vi "expt_controller.vi"() -> ()   [LabVIEW 2019]
uses:
  Quantum Composers 9000 Series/Public/Configure/Configure Chan Mode (Normal).vi
  Quantum Composers 9000 Series/Quantum Composers 9000 Series.lvlib
panel:
  in  "Save condtions":bool=TRUE
  in  "Tab Control":T1(tab)
  in  "Target translation / V":dbl
  in  "Target rotation / V":dbl
  in  "Float / V":dbl
  in  "Q-switch delay / us":dbl
  in  "Delay (rel to gas pulse) / us":dbl
  in  "Gas pulse enable":bool
  in  "Ablation Laser Enable":bool
  in  "stop":bool
  in  "stop 2":bool
  in  "Tab Control 2":enum32{"Ion Optics", "Gas Controls"}(tab)
  in  "Einzel A 1+3 / V":dbl
  in  "Einzel A 2 / V":dbl
  in  "Deceleration Float / V":dbl
  in  "Einzel B 2 / V":dbl
  in  "Def Top / V":dbl
  in  "Def Bottom / V":dbl
  in  "Def Left / V":dbl
  in  "Def Right / V":dbl
  in  "Ref Extraction Sync Source (0:To)":i32(ring)=2 items=["System (To)", "Channel A", "Channel B", "Channel C", "Channel D", "Channel E", "Channel F", "Channel G", "Channel H"]
  in  "MCP":dbl
  in  "R1 / V 2":dbl
  in  "R2 / V":dbl
  in  "Deflection Plate  2 / V 2":dbl
  in  "Deflection Plate  1 / V":dbl
  in  "Einzel C 2 / V":dbl
  in  "Ref Width / us":dbl=1.0 min=1.0 step=1.0
  in  "Ref Delay / us":dbl
  in  "Ref Extraction Enable":bool
  in  "Ref Repeller / V":dbl
  in  "Ref Extractor / V":dbl
  in  "Ref Gnd / V":dbl
  in  "IR Laser Delay / us":dbl=1.0 min=1.0
  in  "IR Laser Q-switch Delay / us":dbl
  in  "IR Laser Sync Source (0:To)":i32(ring)=2 items=["System (To)", "Channel A", "Channel B", "Channel C", "Channel D", "Channel E", "Channel F", "Channel G", "Channel H"]
  in  "IR Laser Enable":bool
  in  "Scope Enable":bool
  in  "Scope Delay / us":dbl format="%#_13g"
  in  "Scope Sync Source (0:To)":i32(ring)=2 items=["System (To)", "Channel A", "Channel B", "Channel C", "Channel D", "Channel E", "Channel F", "Channel G", "Channel H"]
  out "Channel 1 Pressure":cluster{i32[], dbl[]}(graph)
  # "Ablation Laser"
  # "Other Controls"
  # "Einzel Lens A"
  # "Deceleration"
  # "Einzel Lens B"
  # "Decel float determines Einzel B 1/3"
  # "Deflection"
  # "Extraction"
  # "Guidence"
  # "Reflectron"
  # "MCPs"
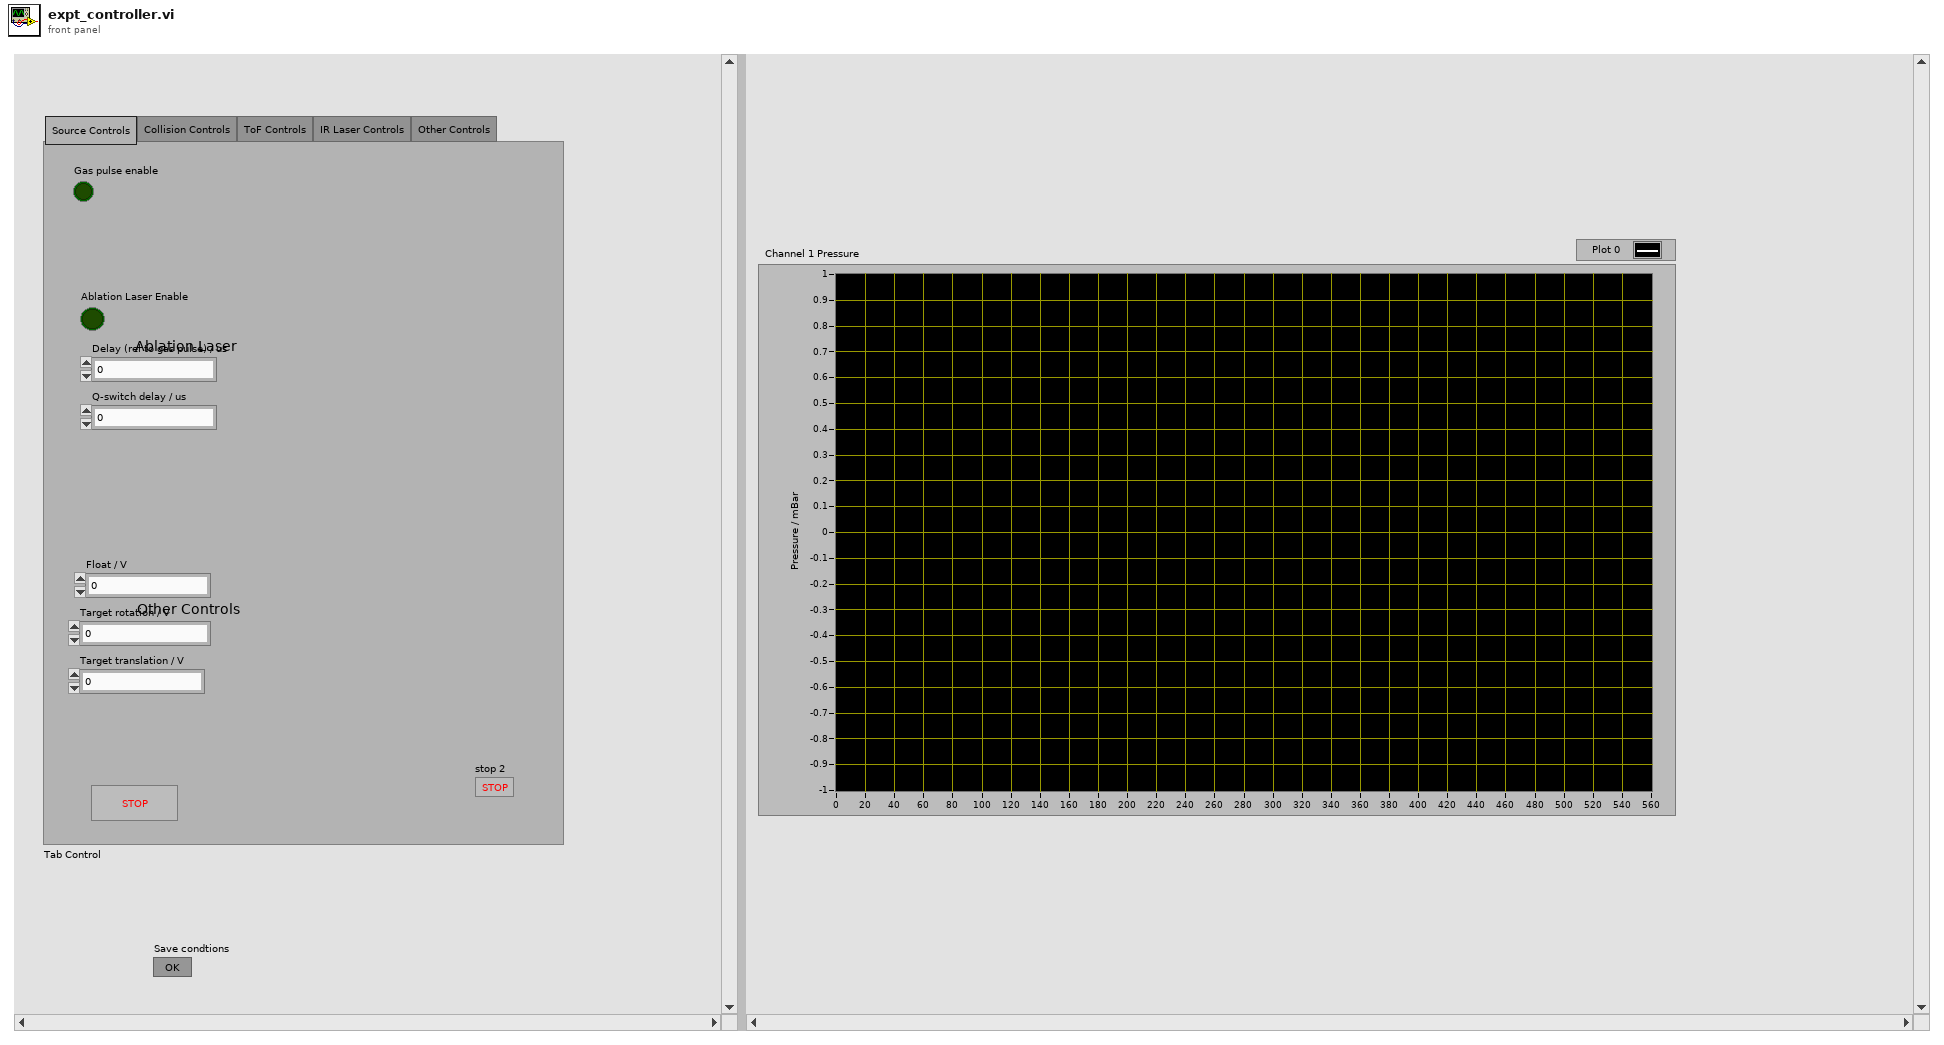
[diagram p1: front panel]
types:
  T1 = enum32{"Source Controls", "Collision Controls", "ToF Controls", "IR Laser Controls", "Other Controls"}
  T2 = cluster{"Ref Extraction Sync Source (0:To)":i32, "Scope Sync Source (0:To)":i32, "IR Laser Sync Source (0:To)":i32, "Gas pulse enable":bool, "Ablation Laser Enable":bool, "Ref Extraction Enable":bool, "Scope Enable":bool, "IR Laser Enable":bool, "Delay (rel to gas pulse) / us":dbl, "Q-switch delay / us":dbl, "Ref Delay / us":dbl, "Scope Delay / us":dbl, "IR Laser Delay / us":dbl, "IR Laser Q-switch Delay / us":dbl, "Ref Width / us":dbl, "Target rotation / V":dbl, "Target translation / V":dbl, "Float / V":dbl, "Einzel A 1+3 / V":dbl, "Einzel A 2 / V":dbl, "Deceleration Float / V":dbl, "Einzel B 2 / V":dbl, "Def Top / V":dbl, "Def Bottom / V":dbl, "Def Left / V":dbl, "Def Right / V":dbl, "Ref Repeller / V":dbl, "Ref Extractor / V ":dbl, "Ref Gnd / V ":dbl, "Einzel C 2 / V":dbl, "Deflection Plate  1 / V":dbl, "Deflection Plate  2 / V 2":dbl, "R1 / V 2":dbl, "R2 / V":dbl, "MCP":dbl}
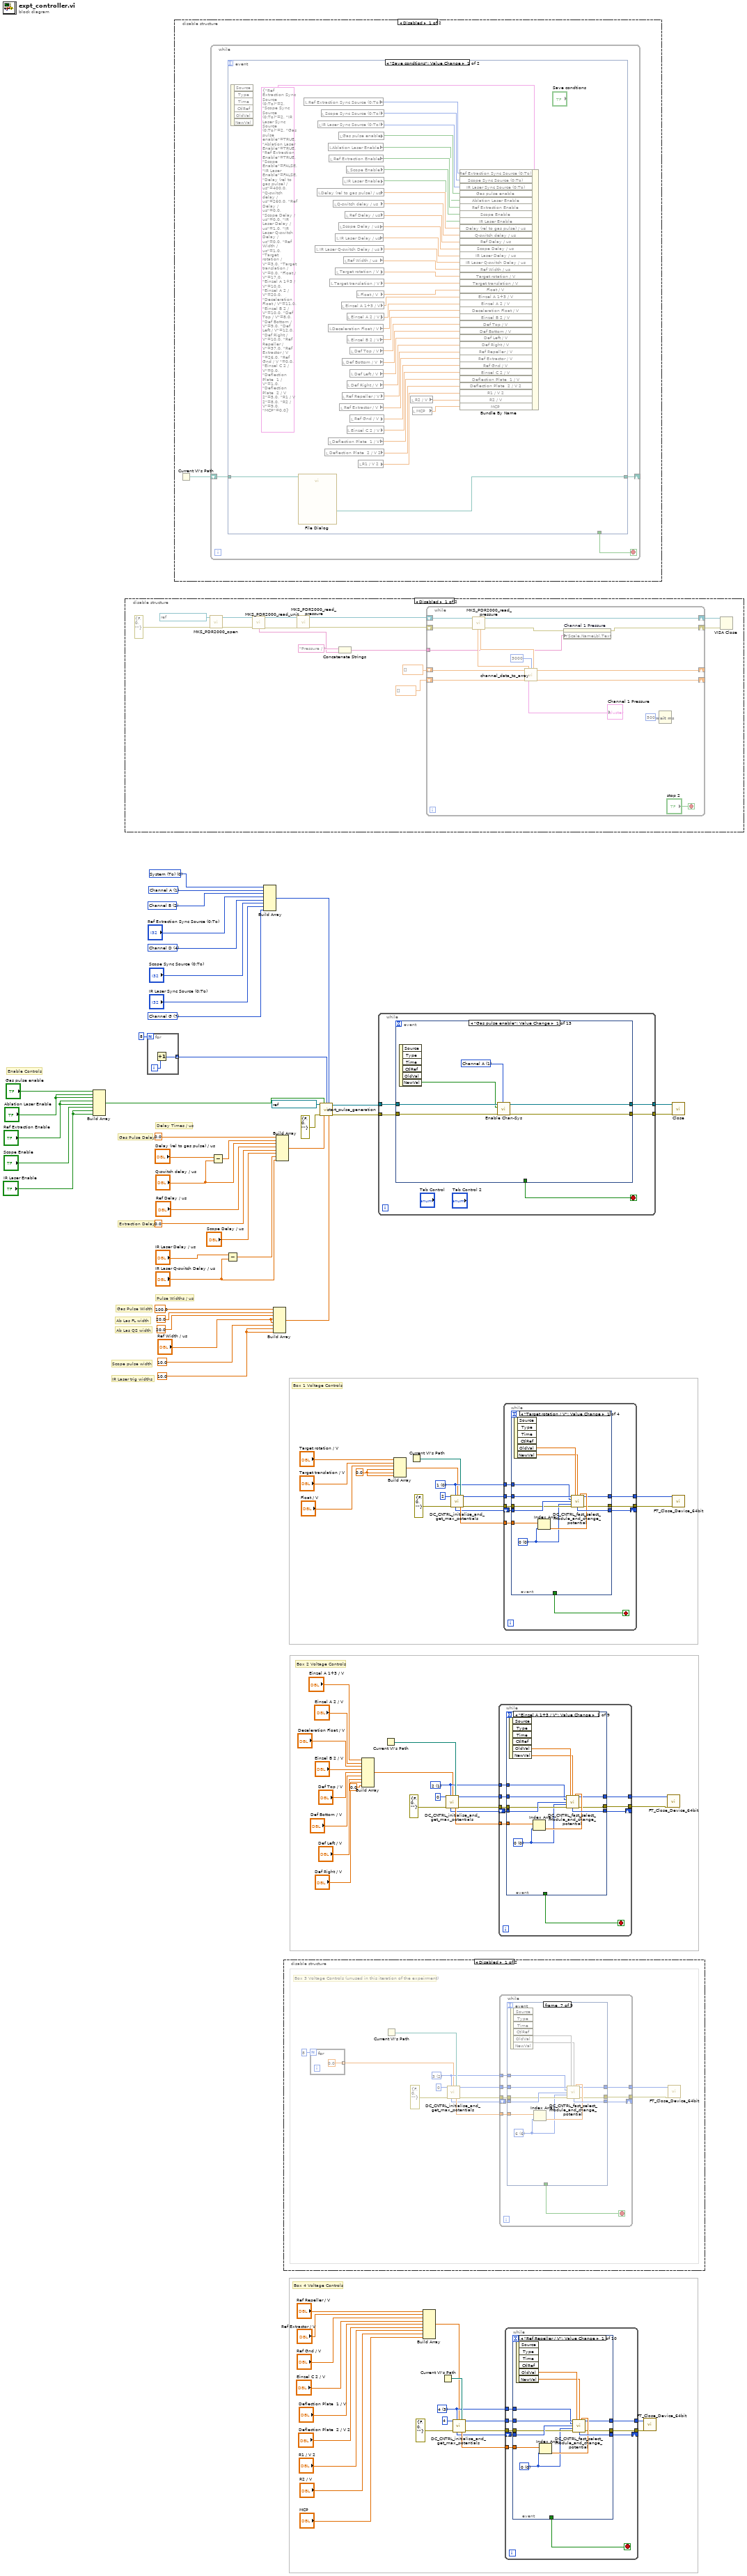
[diagram p0: block diagram]
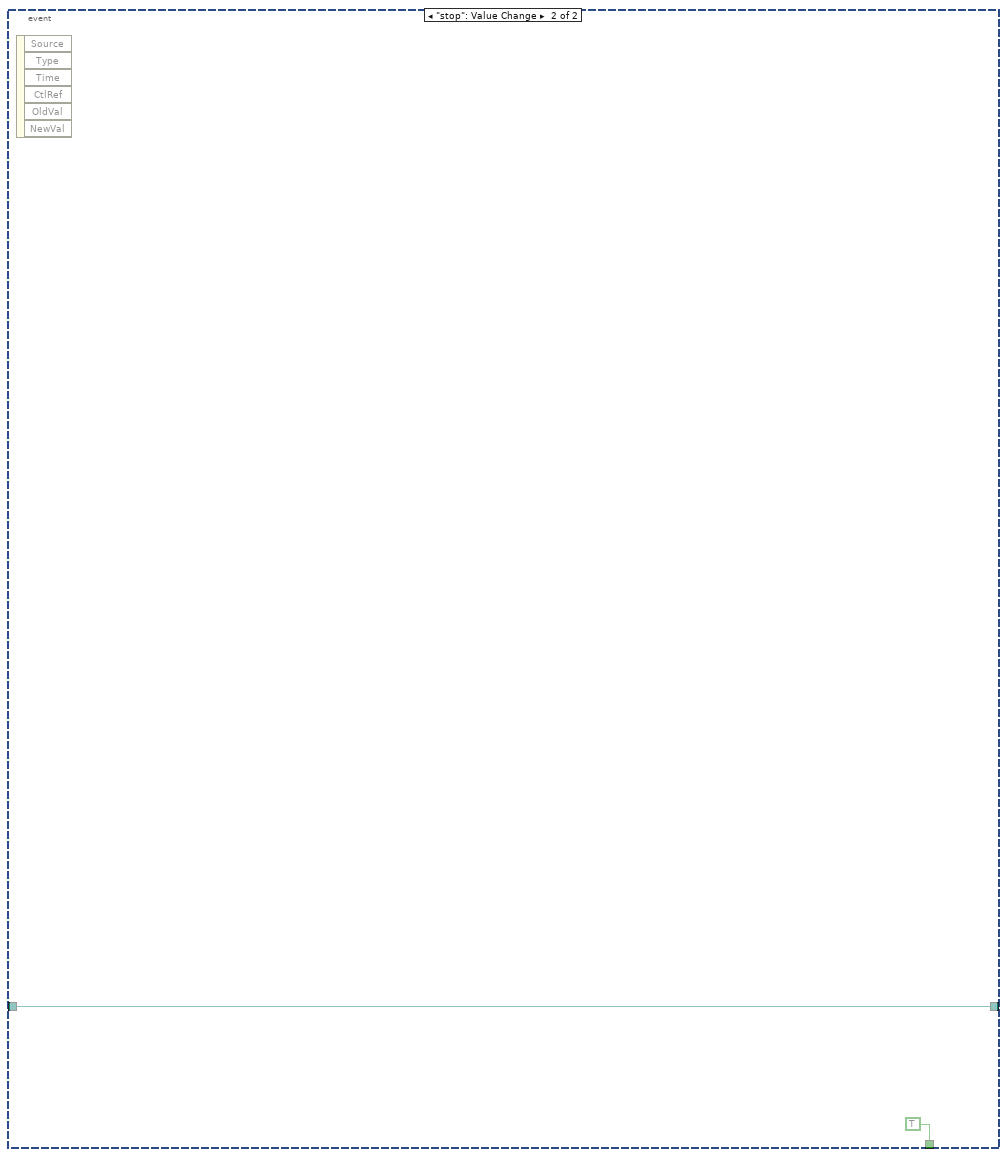
[diagram p2: hidden frame]
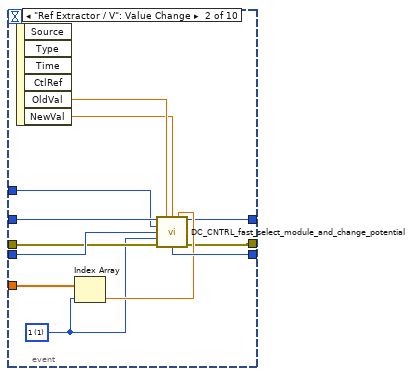
[diagram p5: hidden frame]
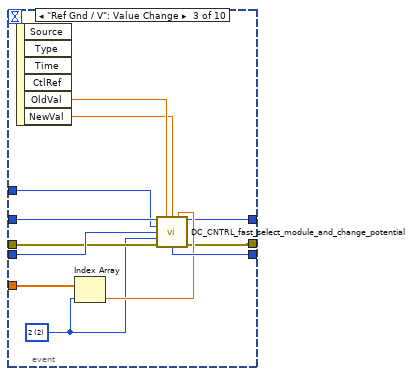
[diagram p6: hidden frame]
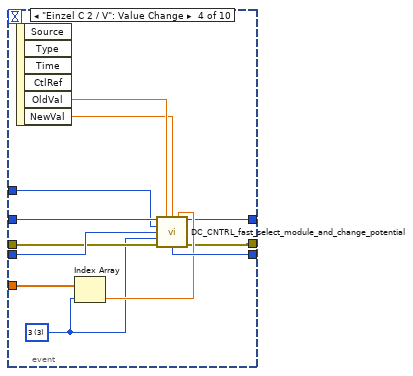
[diagram p7: hidden frame]
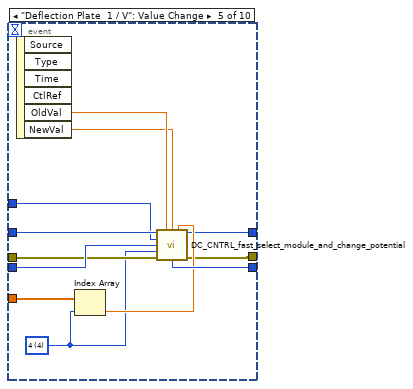
[diagram p8: hidden frame]
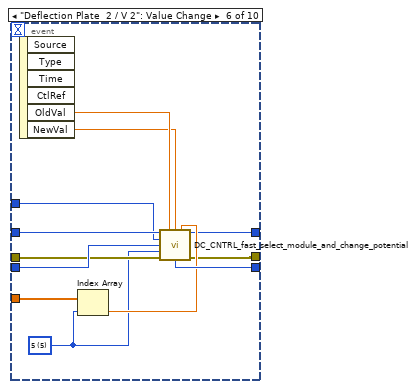
[diagram p9: hidden frame]
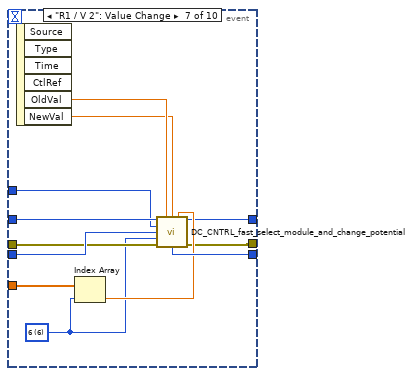
[diagram p10: hidden frame]
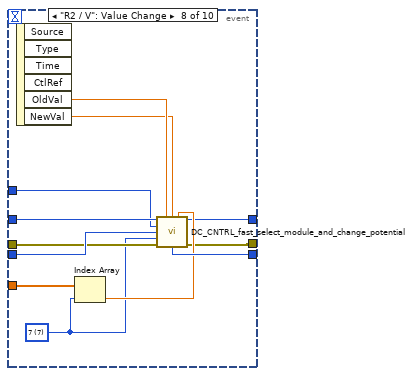
[diagram p11: hidden frame]
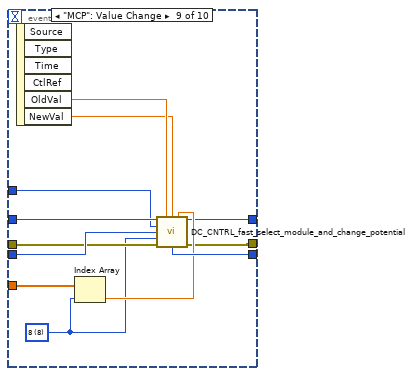
[diagram p12: hidden frame]
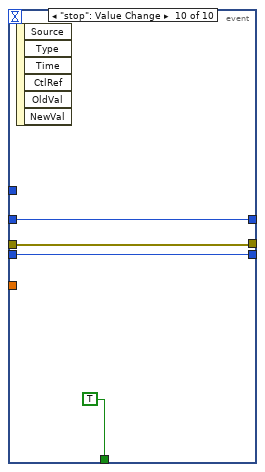
[diagram p13: hidden frame]
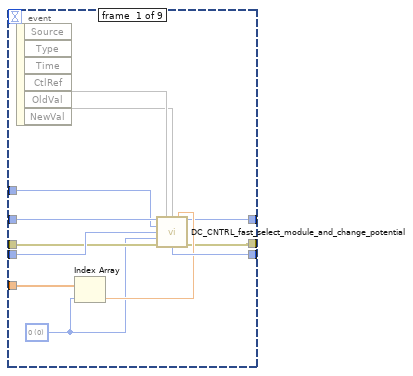
[diagram p14: hidden frame]
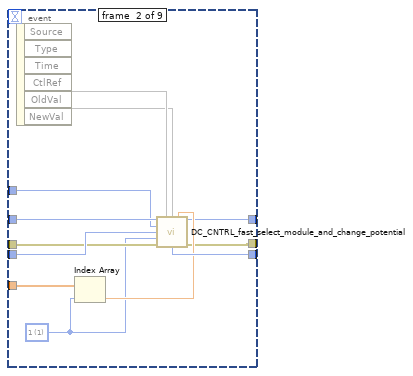
[diagram p15: hidden frame]
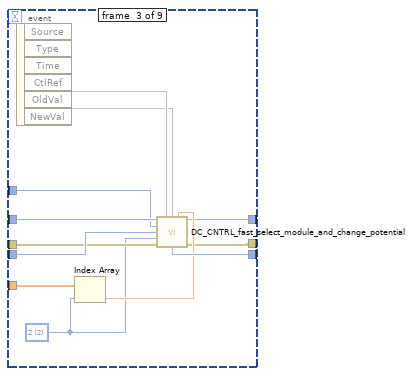
[diagram p16: hidden frame]
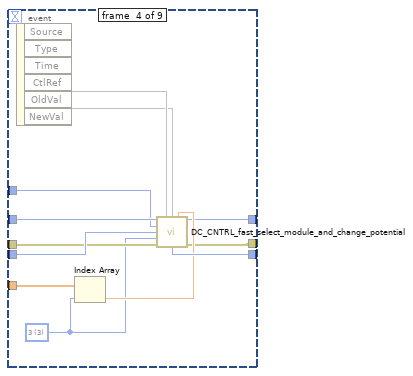
[diagram p17: hidden frame]
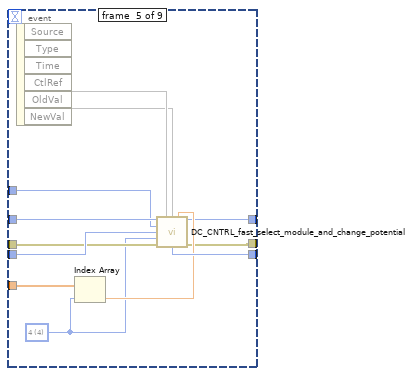
[diagram p18: hidden frame]
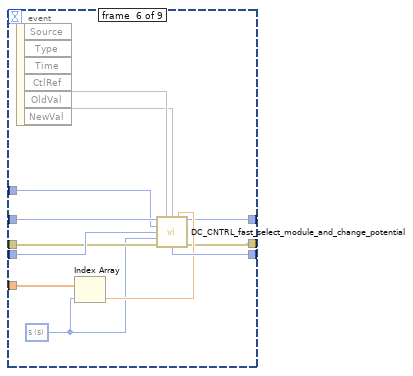
[diagram p19: hidden frame]
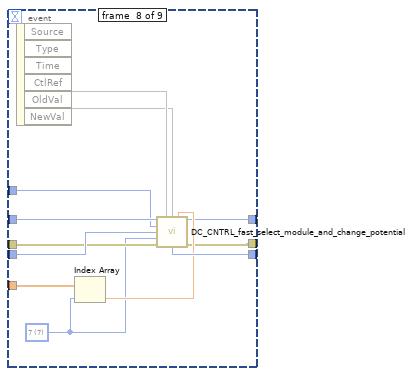
[diagram p20: hidden frame]
diagram:
  w2 = u16 3 items=["1", "2", "3", "4"] ("Box Number")
  w13 = u16 1 items=["1", "2", "3", "4"] ("Box Number")
  w24 = u16 0 items=["1", "2", "3", "4"] ("Box Number")
  w52 = 0.0 ("element")
  w61 = 10.0 ("IR Laser Flashlamp Width / us")
  w73 = 7 items=["System (To)", "Channel A", "Channel B", "Channel C", "Channel D", "Channel E", "Channel F", "Channel G", "Channel H"] ("Sync Source (0:To)")
  w76 = 4 items=["System (To)", "Channel A", "Channel B", "Channel C", "Channel D", "Channel E", "Channel F", "Channel G", "Channel H"] ("Sync Source (0:To)")
  w78 = 2 items=["System (To)", "Channel A", "Channel B", "Channel C", "Channel D", "Channel E", "Channel F", "Channel G", "Channel H"] ("Sync Source (0:To)")
  w79 = 1 items=["System (To)", "Channel A", "Channel B", "Channel C", "Channel D", "Channel E", "Channel F", "Channel G", "Channel H"] ("Sync Source (0:To)")
  w80 = 0 items=["System (To)", "Channel A", "Channel B", "Channel C", "Channel D", "Channel E", "Channel F", "Channel G", "Channel H"] ("Sync Source (0:To)")
  # "Box 4 Voltage Controls"
  # "Box 2 Voltage Controls"
  # "Box 1 Voltage Controls"
  # "IR Laser trig widths"
  # "Scope pulse width"
  # "Enable Controls"
  # "Pulse Widths / us"
  # "Ab Las QS width"
  # "Ab Las FL width"
  # "Gas Pulse Width"
  # "Gas Pulse Delay"
  # "Extraction Delay"
  # "Delay Times / us"
  n1 = Build Array("Gas pulse enable", "Ablation Laser Enable", "Ablation Laser Enable", "Ref Extraction Enable", "Ref Extraction Enable", "Scope Enable", "IR Laser Enable", "IR Laser Enable") -> (w65:bool[])
  n2 = disable-structure shown="Disabled" {
    frame Disabled {
      n3 = call "MKS_PDR2000_open.vi"("error in (no error)"=errorcluster {"status"=FALSE, "code"=0, "source"=""}, "PDR2000 COM port"=refnum<visa-resource-name> "PDR_2000") -> ("error out"=w108:errorcluster, "PDR2000 COM port out"=w109:refnum<visa-resource-name>)  [unwired: 8 in]
      n4 = call "MKS_PDR2000_read_unit.vi"("PDR2000 COM port"=w109, "error in (no error)"=w108) -> ("PDR2000 COM port out"=w105:refnum<visa-resource-name>, "Unit"=w98:string, "error out"=w104:errorcluster)  [unwired: 11 in]
      n5 = call "MKS_PDR2000_read_pressure.vi"("error in (no error)"=w104, "PDR2000 COM port"=w105) -> ("error out"=w102:errorcluster, "PDR2000 COM port out"=w103:refnum<visa-resource-name>)  [unwired: 6 in, 2 out]
      n6 = Concatenate Strings("Pressure / ", w98) -> (w97:string)
      n7 = while {
        shift-right: [w125] -> w107
        shift-left: w103 -> [w127]
        shift-right: [w113] -> w106
        shift-left: w102 -> [w126]
        shift-right: [w122] -> _
        shift-left: dbl[] [] -> [w124]
        shift-right: [w121] -> _
        shift-left: dbl[] [] -> [w123]
        tunnel: w97 -> [w114]
        stop <- "stop 2" stop-if-true
        n8 = call "MKS_PDR2000_read_pressure.vi"("error in (no error)"=w126, "PDR2000 COM port"=w127) -> ("error out"=w115:errorcluster, "PDR2000 COM port out"=w125:refnum<visa-resource-name>, "Channel 2 Pressure"=w119:dbl, "Channel 1 Pressure"=w120:dbl)  [unwired: 6 in]
        n9 = call "channel_data_to_array.vi"("Channel 1 Pressures Array"=w124, "Channel 1 Pressure"=w120, "Max Array Size"=3000, "Channel 2 Pressure"=w119, "Channel 2 Pressures Array"=w123) -> ("Channel 1 Pressures Array Out"=w122:dbl[], "Channel 1 XY data"=→"Channel 1 Pressure":cluster{i32[], dbl[]}, "Channel 2 Pressures Array Out"=w121:dbl[])  [unwired: 7 in, 1 out]
        n10 = property on="Channel 1 Pressure" class="XYGraph (strict)"(error in=w115, "YScale.NameLbl.Text"=w114) -> (error out=w113:errorcluster)  [unwired: 1 in, 1 out]
        n11 = Wait (ms)(milliseconds to wait=u32 500) -> ()  [unwired: 1 out]
      }
      n12 = VISA Close(VISA resource name=w107, error in (no error)=w106) -> ()  [unwired: 1 out]
    }
    frame Enabled {
    }
  }
  n13 = for {
    N: 8 -> [_]
    tunnel: [w128] -> w70 mode=indexing
    i -> [w129]
    n14 = Increment(x=w129) -> (x+1=w128:i32)
  }
  n15 = disable-structure shown="Disabled" {
    frame Disabled {
      n16 = Current VI's Path() -> (path=w130:path)
      n17 = while {
        shift-right: [w132] -> _
        shift-left: w130 -> [w133]
        stop <- w131 stop-if-true
        n18 = event shown="[0] \"Save condtions\": Value Change" {
          selector: _ -> [_ _]
          dyn-events: _ -> [_ _]
          timeout: _ -> [_ _]
          tunnel: w133 -> [w135 w172]
          tunnel: [w134 w172] -> w132
          tunnel: [_ TRUE] -> w131
          event "Save condtions": Value Change {
            n19 = event-data() -> ()  [unwired: 1 in, 6 out]
            n20 = call "File Dialog"("start path"=w135) -> ("selected path"=w134:path)  [unwired: 11 in, 3 out]
            n21 = local read "Ref Extraction Sync Source (0:To)"() -> (w137:i32)
            n22 = local read "IR Laser Q-switch Delay / us"() -> (w150:dbl)
            n23 = local read "Delay (rel to gas pulse) / us"() -> (w145:dbl)
            n24 = local read "IR Laser Sync Source (0:To)"() -> (w139:i32)
            n25 = local read "Scope Sync Source (0:To)"() -> (w138:i32)
            n26 = local read "Deflection Plate  2 / V 2"() -> (w168:dbl)
            n27 = local read "Ablation Laser Enable"() -> (w141:bool)
            n28 = local read "Deceleration Float / V"() -> (w157:dbl)
            n29 = local read "Deflection Plate  1 / V"() -> (w167:dbl)
            n30 = local read "Ref Extraction Enable"() -> (w142:bool)
            n31 = local read "Target translation / V"() -> (w153:dbl)
            n32 = local read "Q-switch delay / us"() -> (w146:dbl)
            n33 = local read "IR Laser Delay / us"() -> (w149:dbl)
            n34 = local read "Target rotation / V"() -> (w152:dbl)
            n35 = local read "Gas pulse enable"() -> (w140:bool)
            n36 = local read "Scope Delay / us"() -> (w148:dbl)
            n37 = local read "Ref Extractor / V"() -> (w164:dbl)
            n38 = local read "Einzel A 1+3 / V"() -> (w155:dbl)
            n39 = local read "Def Bottom / V"() -> (w160:dbl)
            n40 = local read "Ref Repeller / V"() -> (w163:dbl)
            n41 = local read "IR Laser Enable"() -> (w144:bool)
            n42 = local read "Ref Width / us"() -> (w151:dbl)
            n43 = local read "Ref Delay / us"() -> (w147:dbl)
            n44 = local read "Scope Enable"() -> (w143:bool)
            n45 = local read "Einzel A 2 / V"() -> (w156:dbl)
            n46 = local read "Einzel B 2 / V"() -> (w158:dbl)
            n47 = local read "Def Right / V"() -> (w162:dbl)
            n48 = local read "Einzel C 2 / V"() -> (w166:dbl)
            n49 = local read "Def Top / V"() -> (w159:dbl)
            n50 = local read "Def Left / V"() -> (w161:dbl)
            n51 = local read "Ref Gnd / V"() -> (w165:dbl)
            n52 = local read "Float / V"() -> (w154:dbl)
            n53 = local read "R1 / V 2"() -> (w169:dbl)
            n54 = local read "R2 / V"() -> (w170:dbl)
            n55 = local read "MCP"() -> (w171:dbl)
            n56 = Bundle By Name(cluster=T2 {"Ref Extraction Sync Source (0:To)"=2, "Scope Sync Source (0:To)"=2, "IR Laser Sync Source (0:To)"=2, "Gas pulse enable"=TRUE, "Ablation Laser Enable"=TRUE, "Ref Extraction Enable"=TRUE, "Scope Enable"=FALSE, "IR Laser Enable"=FALSE, "Delay (rel to gas pulse) / us"=400.0, "Q-switch delay / us"=260.0, "Ref Delay / us"=0.0, "Scope Delay / us"=0.0, "IR Laser Delay / us"=1.0, "IR Laser Q-switch Delay / us"=0.0, "Ref Width / us"=1.0, "Target rotation / V"=3.0, "Target translation / V"=0.0, "Float / V"=17.0, "Einzel A 1+3 / V"=10.0, "Einzel A 2 / V"=20.0, "Deceleration Float / V"=11.0, "Einzel B 2 / V"=10.0, "Def Top / V"=8.0, "Def Bottom / V"=9.0, "Def Left / V"=12.0, "Def Right / V"=10.0, "Ref Repeller / V"=37.0, "Ref Extractor / V "=26.0, "Ref Gnd / V "=0.0, "Einzel C 2 / V"=0.0, "Deflection Plate  1 / V"=1.0, "Deflection Plate  2 / V 2"=5.0, "R1 / V 2"=8.0, "R2 / V"=9.0, "MCP"=0.0} ("input cluster"), "Ref Extraction Sync Source (0:To)"=w137, "Scope Sync Source (0:To)"=w138, "IR Laser Sync Source (0:To)"=w139, "Gas pulse enable"=w140, "Ablation Laser Enable"=w141, "Ref Extraction Enable"=w142, "Scope Enable"=w143, "IR Laser Enable"=w144, "Delay (rel to gas pulse) / us"=w145, "Q-switch delay / us"=w146, "Ref Delay / us"=w147, "Scope Delay / us"=w148, "IR Laser Delay / us"=w149, "IR Laser Q-switch Delay / us"=w150, "Ref Width / us"=w151, "Target rotation / V"=w152, "Target translation / V"=w153, "Float / V"=w154, "Einzel A 1+3 / V"=w155, "Einzel A 2 / V"=w156, "Deceleration Float / V"=w157, "Einzel B 2 / V"=w158, "Def Top / V"=w159, "Def Bottom / V"=w160, "Def Left / V"=w161, "Def Right / V"=w162, "Ref Repeller / V"=w163, "Ref Extractor / V"=w164, "Ref Gnd / V"=w165, "Einzel C 2 / V"=w166, "Deflection Plate  1 / V"=w167, "Deflection Plate  2 / V 2"=w168, "R1 / V 2"=w169, "R2 / V"=w170, "MCP"=w171) -> ()  [unwired: 1 out]
          }
          event "stop": Value Change {
            n57 = event-data() -> ()  [unwired: 1 in, 6 out]
          }
        }
      }
    }
    frame Enabled {
    }
  }
  n58 = Subtract(x="Delay (rel to gas pulse) / us", y="Q-switch delay / us") -> (x-y=w94:dbl)
  n59 = Subtract(x="IR Laser Delay / us", y="IR Laser Q-switch Delay / us") -> (x-y=w58:dbl)
  n60 = Build Array(w80, w79, w78, "Ref Extraction Sync Source (0:To)", w76, "Scope Sync Source (0:To)", "IR Laser Sync Source (0:To)", w73) -> (w72:i32[])
  n61 = Build Array(100.0, 20.0, 20.0, "Ref Width / us", "Ref Width / us", 10.0, w61, w61) -> (w83:dbl[])
  n62 = Build Array(0.0, w94, "Q-switch delay / us", "Ref Delay / us", 0.0, "Scope Delay / us", w58, "IR Laser Q-switch Delay / us") -> (w89:dbl[])
  n63 = disable-structure shown="Disabled" {
    frame Disabled {
      w175 = u16 2 items=["1", "2", "3", "4"] ("Box Number")
      # "Box 3 Voltage Controls (unused in this iteration of the expeirment)"
      n64 = for {
        N: 8 -> [_]
        tunnel: [0.0] -> w174 mode=indexing
      }
      n65 = Current VI's Path() -> (path=w182:path)
      n66 = call "DC_CNTRL_initialise_and_get_max_potentials.vi"("Device Index"=u32 0, "Box Number"=w175, "Input Potentials"=w174, "Current VI Path"=w182, "error in (no error)"=errorcluster {"status"=FALSE, "code"=0, "source"=""}) -> ("Handle out"=w181:u64, "Current Module"=w179:i32, "Max Range Array"=w180:dbl[], "error out"=w178:errorcluster)  [unwired: 7 in]
      n67 = while {
        tunnel: w181 -> [w194]
        tunnel: w180 -> [w193]
        tunnel: w178 -> [w191]
        shift-right: [w190] -> _
        shift-left: w179 -> [w192]
        tunnel: [w189] -> w177
        tunnel: [w188] -> w176
        tunnel: w175 -> [w186]
        stop <- w187 stop-if-true
        n68 = event {
          selector: _ -> [_ _ _ _ _ _ _ _ _]
          dyn-events: _ -> [_ _ _ _ _ _ _ _ _]
          timeout: _ -> [_ _ _ _ _ _ _ _ _]
          tunnel: w194 -> [w206 w218 w230 w242 w254 w266 w278 w290 w293]
          tunnel: w193 -> [w203 w215 w227 w239 w251 w263 w275 w287 _]
          tunnel: w192 -> [w202 w214 w226 w238 w250 w262 w274 w286 w291]
          tunnel: w191 -> [w201 w213 w225 w237 w249 w261 w273 w285 w292]
          tunnel: [w200 w212 w224 w236 w248 w260 w272 w284 w291] -> w190
          tunnel: [w197 w209 w221 w233 w245 w257 w269 w281 w293] -> w189
          tunnel: [w196 w208 w220 w232 w244 w256 w268 w280 w292] -> w188
          tunnel: [_ _ _ _ _ _ _ _ TRUE] -> w187
          tunnel: w186 -> [w195 w207 w219 w231 w243 w255 w267 w279 _]
          event #0 {
            w198 = u16 0 items=["0", "1", "2", "3", "4", "5", "6", "7"] ("Desired Module Number")
            n69 = event-data() -> ("OldVal"=w205, "NewVal"=w204)  [unwired: 1 in, 4 out]
            n70 = Index Array(array=w203, index=w198) -> (element=w199:dbl)
            n71 = call "DC_CNTRL_fast_select_module_and_change_potential.vi"("Handle in"=w206, "Current Potential (V)"=w205, "Target Potential (V)"=w204, "Max Potential (V)"=w199, "Box Number"=w195, "Current Module Number"=w202, "Desired Module Number"=w198, "error in (no error)"=w201) -> ("Handle out"=w197:u64, "Current Module Number Out"=w200:u16, "error out"=w196:errorcluster)  [unwired: 5 in]
          }
          event #1 {
            w210 = u16 1 items=["0", "1", "2", "3", "4", "5", "6", "7"] ("Desired Module Number")
            n72 = event-data() -> ("OldVal"=w217, "NewVal"=w216)  [unwired: 1 in, 4 out]
            n73 = Index Array(array=w215, index=w210) -> (element=w211:dbl)
            n74 = call "DC_CNTRL_fast_select_module_and_change_potential.vi"("Handle in"=w218, "Current Potential (V)"=w217, "Target Potential (V)"=w216, "Max Potential (V)"=w211, "Box Number"=w207, "Current Module Number"=w214, "Desired Module Number"=w210, "error in (no error)"=w213) -> ("Handle out"=w209:u64, "Current Module Number Out"=w212:u16, "error out"=w208:errorcluster)  [unwired: 5 in]
          }
          event #2 {
            w222 = u16 2 items=["0", "1", "2", "3", "4", "5", "6", "7"] ("Desired Module Number")
            n75 = event-data() -> ("OldVal"=w229, "NewVal"=w228)  [unwired: 1 in, 4 out]
            n76 = Index Array(array=w227, index=w222) -> (element=w223:dbl)
            n77 = call "DC_CNTRL_fast_select_module_and_change_potential.vi"("Handle in"=w230, "Current Potential (V)"=w229, "Target Potential (V)"=w228, "Max Potential (V)"=w223, "Box Number"=w219, "Current Module Number"=w226, "Desired Module Number"=w222, "error in (no error)"=w225) -> ("Handle out"=w221:u64, "Current Module Number Out"=w224:u16, "error out"=w220:errorcluster)  [unwired: 5 in]
          }
          event #3 {
            w234 = u16 3 items=["0", "1", "2", "3", "4", "5", "6", "7"] ("Desired Module Number")
            n78 = event-data() -> ("OldVal"=w241, "NewVal"=w240)  [unwired: 1 in, 4 out]
            n79 = Index Array(array=w239, index=w234) -> (element=w235:dbl)
            n80 = call "DC_CNTRL_fast_select_module_and_change_potential.vi"("Handle in"=w242, "Current Potential (V)"=w241, "Target Potential (V)"=w240, "Max Potential (V)"=w235, "Box Number"=w231, "Current Module Number"=w238, "Desired Module Number"=w234, "error in (no error)"=w237) -> ("Handle out"=w233:u64, "Current Module Number Out"=w236:u16, "error out"=w232:errorcluster)  [unwired: 5 in]
          }
          event #4 {
            w246 = u16 4 items=["0", "1", "2", "3", "4", "5", "6", "7"] ("Desired Module Number")
            n81 = event-data() -> ("OldVal"=w253, "NewVal"=w252)  [unwired: 1 in, 4 out]
            n82 = Index Array(array=w251, index=w246) -> (element=w247:dbl)
            n83 = call "DC_CNTRL_fast_select_module_and_change_potential.vi"("Handle in"=w254, "Current Potential (V)"=w253, "Target Potential (V)"=w252, "Max Potential (V)"=w247, "Box Number"=w243, "Current Module Number"=w250, "Desired Module Number"=w246, "error in (no error)"=w249) -> ("Handle out"=w245:u64, "Current Module Number Out"=w248:u16, "error out"=w244:errorcluster)  [unwired: 5 in]
          }
          event #5 {
            w258 = u16 5 items=["0", "1", "2", "3", "4", "5", "6", "7"] ("Desired Module Number")
            n84 = event-data() -> ("OldVal"=w265, "NewVal"=w264)  [unwired: 1 in, 4 out]
            n85 = Index Array(array=w263, index=w258) -> (element=w259:dbl)
            n86 = call "DC_CNTRL_fast_select_module_and_change_potential.vi"("Handle in"=w266, "Current Potential (V)"=w265, "Target Potential (V)"=w264, "Max Potential (V)"=w259, "Box Number"=w255, "Current Module Number"=w262, "Desired Module Number"=w258, "error in (no error)"=w261) -> ("Handle out"=w257:u64, "Current Module Number Out"=w260:u16, "error out"=w256:errorcluster)  [unwired: 5 in]
          }
          event #6 {
            w270 = u16 6 items=["0", "1", "2", "3", "4", "5", "6", "7"] ("Desired Module Number")
            n87 = event-data() -> ("OldVal"=w277, "NewVal"=w276)  [unwired: 1 in, 4 out]
            n88 = Index Array(array=w275, index=w270) -> (element=w271:dbl)
            n89 = call "DC_CNTRL_fast_select_module_and_change_potential.vi"("Handle in"=w278, "Current Potential (V)"=w277, "Target Potential (V)"=w276, "Max Potential (V)"=w271, "Box Number"=w267, "Current Module Number"=w274, "Desired Module Number"=w270, "error in (no error)"=w273) -> ("Handle out"=w269:u64, "Current Module Number Out"=w272:u16, "error out"=w268:errorcluster)  [unwired: 5 in]
          }
          event #7 {
            w282 = u16 7 items=["0", "1", "2", "3", "4", "5", "6", "7"] ("Desired Module Number")
            n90 = event-data() -> ("OldVal"=w289, "NewVal"=w288)  [unwired: 1 in, 4 out]
            n91 = Index Array(array=w287, index=w282) -> (element=w283:dbl)
            n92 = call "DC_CNTRL_fast_select_module_and_change_potential.vi"("Handle in"=w290, "Current Potential (V)"=w289, "Target Potential (V)"=w288, "Max Potential (V)"=w283, "Box Number"=w279, "Current Module Number"=w286, "Desired Module Number"=w282, "error in (no error)"=w285) -> ("Handle out"=w281:u64, "Current Module Number Out"=w284:u16, "error out"=w280:errorcluster)  [unwired: 5 in]
          }
          event #8 {
            n93 = event-data() -> ()  [unwired: 1 in, 6 out]
          }
        }
      }
      n94 = call "FT_Close_Device_64bit.vi"("Handle"=w177, "error in (no error)"=w176) -> ()  [unwired: 12 in, 2 out]
    }
    frame Enabled {
    }
  }
  n95 = call "start_pulse_generation.vi"("VISA resource name"=refnum<visa-resource-name> "QC9528_1", "Enabled array"=w65, "Channel Array"=w70, "Sync source array"=w72, "error in (no error)"=errorcluster {"status"=FALSE, "code"=0, "source"=""}, "Delays array"=w89, "Widths array"=w83) -> ("VISA resource name out"=w64:refnum<visa-resource-name>, "error out"=w63:errorcluster)  [unwired: 7 in]
  n96 = Build Array("Einzel A 1+3 / V", "Einzel A 2 / V", "Deceleration Float / V", "Einzel B 2 / V", "Def Top / V", "Def Bottom / V", "Def Left / V", "Def Right / V", 0.0 ("element")) -> (w12:dbl[])
  n97 = while {
    tunnel: w64 -> [w300]
    tunnel: w63 -> [w299]
    tunnel: [w298] -> w57
    tunnel: [w297] -> w56
    stop <- w296 stop-if-true
    n98 = event shown="[0] \"Gas pulse enable\": Value Change" {
      selector: _ -> [_ _ _ _ _ _ _ _ _ _ _ _ _]
      dyn-events: _ -> [_ _ _ _ _ _ _ _ _ _ _ _ _]
      timeout: _ -> [_ _ _ _ _ _ _ _ _ _ _ _ _]
      tunnel: w300 -> [w306 w312 w321 w330 w340 w347 w354 w361 w377 w391 w406 w416 w418]
      tunnel: w299 -> [w305 w311 w320 w329 w339 w345 w352 w359 w376 w390 w405 w415 w417]
      tunnel: [w302 w308 w317 w326 w336 w346 w353 w360 w371 w386 w401 w414 w418] -> w298
      tunnel: [w301 w307 w316 w325 w335 w344 w351 w358 w370 w385 w400 w413 w417] -> w297
      tunnel: [_ _ _ _ FALSE FALSE FALSE FALSE FALSE FALSE FALSE FALSE TRUE] -> w296
      event "Gas pulse enable": Value Change {
        w303 = 1 items=["System (To)", "Channel A", "Channel B", "Channel C", "Channel D", "Channel E", "Channel F", "Channel G", "Channel H"] ("Channel (1:Chan A)")
        n99 = event-data() -> ("NewVal"=w304:bool)  [unwired: 1 in, 5 out]
        n100 = call "Enable Chan-Sys.vi"("Channel (1:Chan A)"=w303, "error in (no error)"=w305, "State (T:Enabled)"=w304, "VISA resource name"=w306) -> ("error out"=w301:errorcluster, "VISA resource name out"=w302:refnum<visa-resource-name>)  [unwired: 6 in]
      }
      event "Scope Enable": Value Change {
        w309 = 6 items=["System (To)", "Channel A", "Channel B", "Channel C", "Channel D", "Channel E", "Channel F", "Channel G", "Channel H"] ("Channel (1:Chan A)")
        n101 = event-data() -> ("NewVal"=w310:bool)  [unwired: 1 in, 5 out]
        n102 = call "Enable Chan-Sys.vi"("Channel (1:Chan A)"=w309, "error in (no error)"=w311, "State (T:Enabled)"=w310, "VISA resource name"=w312) -> ("error out"=w307:errorcluster, "VISA resource name out"=w308:refnum<visa-resource-name>)  [unwired: 6 in]
      }
      event "Ablation Laser Enable": Value Change {
        w313 = 3 items=["System (To)", "Channel A", "Channel B", "Channel C", "Channel D", "Channel E", "Channel F", "Channel G", "Channel H"] ("Channel (1:Chan A)")
        w314 = 2 items=["System (To)", "Channel A", "Channel B", "Channel C", "Channel D", "Channel E", "Channel F", "Channel G", "Channel H"] ("Channel (1:Chan A)")
        n103 = event-data() -> ("NewVal"=w315:bool)  [unwired: 1 in, 5 out]
        n104 = call "Enable Chan-Sys.vi"("Channel (1:Chan A)"=w314, "error in (no error)"=w320, "State (T:Enabled)"=w315, "VISA resource name"=w321) -> ("error out"=w318:errorcluster, "VISA resource name out"=w319:refnum<visa-resource-name>)  [unwired: 6 in]
        n105 = call "Enable Chan-Sys.vi"("Channel (1:Chan A)"=w313, "error in (no error)"=w318, "State (T:Enabled)"=w315, "VISA resource name"=w319) -> ("error out"=w316:errorcluster, "VISA resource name out"=w317:refnum<visa-resource-name>)  [unwired: 6 in]
      }
      event "Ref Extraction Enable": Value Change {
        w322 = 5 items=["System (To)", "Channel A", "Channel B", "Channel C", "Channel D", "Channel E", "Channel F", "Channel G", "Channel H"] ("Channel (1:Chan A)")
        w323 = 4 items=["System (To)", "Channel A", "Channel B", "Channel C", "Channel D", "Channel E", "Channel F", "Channel G", "Channel H"] ("Channel (1:Chan A)")
        n106 = event-data() -> ("NewVal"=w324:bool)  [unwired: 1 in, 5 out]
        n107 = call "Enable Chan-Sys.vi"("Channel (1:Chan A)"=w323, "error in (no error)"=w329, "State (T:Enabled)"=w324, "VISA resource name"=w330) -> ("error out"=w327:errorcluster, "VISA resource name out"=w328:refnum<visa-resource-name>)  [unwired: 6 in]
        n108 = call "Enable Chan-Sys.vi"("Channel (1:Chan A)"=w322, "error in (no error)"=w327, "State (T:Enabled)"=w324, "VISA resource name"=w328) -> ("error out"=w325:errorcluster, "VISA resource name out"=w326:refnum<visa-resource-name>)  [unwired: 6 in]
      }
      event "IR Laser Enable": Value Change {
        w332 = 8 items=["System (To)", "Channel A", "Channel B", "Channel C", "Channel D", "Channel E", "Channel F", "Channel G", "Channel H"] ("Channel (1:Chan A)")
        w333 = 7 items=["System (To)", "Channel A", "Channel B", "Channel C", "Channel D", "Channel E", "Channel F", "Channel G", "Channel H"] ("Channel (1:Chan A)")
        n109 = event-data() -> ("NewVal"=w334:bool)  [unwired: 1 in, 5 out]
        n110 = call "Enable Chan-Sys.vi"("Channel (1:Chan A)"=w333, "error in (no error)"=w339, "State (T:Enabled)"=w334, "VISA resource name"=w340) -> ("error out"=w337:errorcluster, "VISA resource name out"=w338:refnum<visa-resource-name>)  [unwired: 6 in]
        n111 = call "Enable Chan-Sys.vi"("Channel (1:Chan A)"=w332, "error in (no error)"=w337, "State (T:Enabled)"=w334, "VISA resource name"=w338) -> ("error out"=w335:errorcluster, "VISA resource name out"=w336:refnum<visa-resource-name>)  [unwired: 6 in]
      }
      event "Ref Extraction Sync Source (0:To)": Value Change {
        w343 = 4 items=["Channel A"=1, "Channel B"=2, "Channel C"=3, "Channel D"=4, "Channel E"=5, "Channel F"=6, "Channel G"=7, "Channel H"=8] ("Channel (1:Chan A)")
        n112 = event-data() -> ("NewVal"=w342:i32)  [unwired: 1 in, 5 out]
        n113 = call "Configure Chan Input.vi"("Channel (1:Chan A)"=w343, "error in (no error)"=w345, "Sync Source (0:To)"=w342, "VISA resource name"=w347) -> ("error out"=w344:errorcluster, "VISA resource name out"=w346:refnum<visa-resource-name>)  [unwired: 6 in]
      }
      event "Scope Sync Source (0:To)": Value Change {
        w350 = 6 items=["Channel A"=1, "Channel B"=2, "Channel C"=3, "Channel D"=4, "Channel E"=5, "Channel F"=6, "Channel G"=7, "Channel H"=8] ("Channel (1:Chan A)")
        n114 = event-data() -> ("NewVal"=w349:i32)  [unwired: 1 in, 5 out]
        n115 = call "Configure Chan Input.vi"("Channel (1:Chan A)"=w350, "error in (no error)"=w352, "Sync Source (0:To)"=w349, "VISA resource name"=w354) -> ("error out"=w351:errorcluster, "VISA resource name out"=w353:refnum<visa-resource-name>)  [unwired: 6 in]
      }
      event "IR Laser Sync Source (0:To)": Value Change {
        w357 = 7 items=["Channel A"=1, "Channel B"=2, "Channel C"=3, "Channel D"=4, "Channel E"=5, "Channel F"=6, "Channel G"=7, "Channel H"=8] ("Channel (1:Chan A)")
        n116 = event-data() -> ("NewVal"=w356:i32)  [unwired: 1 in, 5 out]
        n117 = call "Configure Chan Input.vi"("Channel (1:Chan A)"=w357, "error in (no error)"=w359, "Sync Source (0:To)"=w356, "VISA resource name"=w361) -> ("error out"=w358:errorcluster, "VISA resource name out"=w360:refnum<visa-resource-name>)  [unwired: 6 in]
      }
      event "Delay (rel to gas pulse) / us", "Q-switch delay / us": Value Change {
        w372 = 3 items=["Channel A"=1, "Channel B"=2, "Channel C"=3, "Channel D"=4, "Channel E"=5, "Channel F"=6, "Channel G"=7, "Channel H"=8] ("Channel (1:Chan A)")
        w375 = 2 items=["Channel A"=1, "Channel B"=2, "Channel C"=3, "Channel D"=4, "Channel E"=5, "Channel F"=6, "Channel G"=7, "Channel H"=8] ("Channel (1:Chan A)")
        n118 = event-data() -> ()  [unwired: 1 in, 6 out]
        n119 = local read "Delay (rel to gas pulse) / us"() -> (w367:dbl)
        n120 = local read "Q-switch delay / us"() -> (w366:dbl)
        n121 = call "us_s_converter.vi"("Time / us"=20.0) -> ("Time / s"=w363:dbl)  [unwired: 4 in]
        n122 = Subtract(x=w367, y=w366) -> (x-y=w365:dbl)
        n123 = call "us_s_converter.vi"("Time / us"=w365) -> ("Time / s"=w364:dbl)  [unwired: 4 in]
        n124 = call-poly "Configure Chan Mode.vi"("Width (10 msec)"=w363, "Delay (10 msec)"=w364, "Channel (1:Chan A)"=w375, "error in (no error)"=w376, "VISA resource name"=w377) -> ("error out"=w373:errorcluster, "VISA resource name out"=w374:refnum<visa-resource-name>)  [unwired: 5 in]
        n125 = call "us_s_converter.vi"("Time / us"=w366) -> ("Time / s"=w369:dbl)  [unwired: 4 in]
        n126 = call-poly "Configure Chan Mode.vi"("Width (10 msec)"=w363, "Delay (10 msec)"=w369, "Channel (1:Chan A)"=w372, "error in (no error)"=w373, "VISA resource name"=w374) -> ("error out"=w370:errorcluster, "VISA resource name out"=w371:refnum<visa-resource-name>)  [unwired: 5 in]
      }
      event "Ref Delay / us", "Ref Width / us": Value Change {
        w384 = 5 items=["Channel A"=1, "Channel B"=2, "Channel C"=3, "Channel D"=4, "Channel E"=5, "Channel F"=6, "Channel G"=7, "Channel H"=8] ("Channel (1:Chan A)")
        w389 = 4 items=["Channel A"=1, "Channel B"=2, "Channel C"=3, "Channel D"=4, "Channel E"=5, "Channel F"=6, "Channel G"=7, "Channel H"=8] ("Channel (1:Chan A)")
        n127 = event-data() -> ()  [unwired: 1 in, 6 out]
        n128 = local read "Ref Delay / us"() -> (w381:dbl)
        n129 = local read "Ref Width / us"() -> (w382:dbl)
        n130 = call "us_s_converter.vi"("Time / us"=w382) -> ("Time / s"=w379:dbl)  [unwired: 4 in]
        n131 = call "us_s_converter.vi"("Time / us"=w381) -> ("Time / s"=w380:dbl)  [unwired: 4 in]
        n132 = call-poly "Configure Chan Mode.vi"("Width (10 msec)"=w379, "Delay (10 msec)"=w380, "Channel (1:Chan A)"=w389, "error in (no error)"=w390, "VISA resource name"=w391) -> ("error out"=w387:errorcluster, "VISA resource name out"=w388:refnum<visa-resource-name>)  [unwired: 5 in]
        n133 = call-poly "Configure Chan Mode.vi"("Width (10 msec)"=w379, "Delay (10 msec)"=0.0, "Channel (1:Chan A)"=w384, "error in (no error)"=w387, "VISA resource name"=w388) -> ("error out"=w385:errorcluster, "VISA resource name out"=w386:refnum<visa-resource-name>)  [unwired: 5 in]
      }
      event "IR Laser Delay / us", "IR Laser Q-switch Delay / us": Value Change {
        w399 = 8 items=["Channel A"=1, "Channel B"=2, "Channel C"=3, "Channel D"=4, "Channel E"=5, "Channel F"=6, "Channel G"=7, "Channel H"=8] ("Channel (1:Chan A)")
        w404 = 7 items=["Channel A"=1, "Channel B"=2, "Channel C"=3, "Channel D"=4, "Channel E"=5, "Channel F"=6, "Channel G"=7, "Channel H"=8] ("Channel (1:Chan A)")
        n134 = event-data() -> ()  [unwired: 1 in, 6 out]
        n135 = local read "IR Laser Q-switch Delay / us"() -> (w398:dbl)
        n136 = local read "IR Laser Delay / us"() -> (w397:dbl)
        n137 = call "us_s_converter.vi"("Time / us"=10.0) -> ("Time / s"=w393:dbl)  [unwired: 4 in]
        n138 = call "us_s_converter.vi"("Time / us"=w397) -> ("Time / s"=w396:dbl)  [unwired: 4 in]
        n139 = call-poly "Configure Chan Mode.vi"("Width (10 msec)"=w393, "Delay (10 msec)"=w396, "Channel (1:Chan A)"=w404, "error in (no error)"=w405, "VISA resource name"=w406) -> ("error out"=w402:errorcluster, "VISA resource name out"=w403:refnum<visa-resource-name>)  [unwired: 5 in]
        n140 = call "us_s_converter.vi"("Time / us"=w398) -> ("Time / s"=w395:dbl)  [unwired: 4 in]
        n141 = call-poly "Configure Chan Mode.vi"("Width (10 msec)"=w393, "Delay (10 msec)"=w395, "Channel (1:Chan A)"=w399, "error in (no error)"=w402, "VISA resource name"=w403) -> ("error out"=w400:errorcluster, "VISA resource name out"=w401:refnum<visa-resource-name>)  [unwired: 5 in]
      }
      event "Scope Delay / us": Value Change {
        w412 = 6 items=["Channel A"=1, "Channel B"=2, "Channel C"=3, "Channel D"=4, "Channel E"=5, "Channel F"=6, "Channel G"=7, "Channel H"=8] ("Channel (1:Chan A)")
        n142 = event-data() -> ()  [unwired: 1 in, 6 out]
        n143 = local read "Scope Delay / us"() -> (w411:dbl)
        n144 = call "us_s_converter.vi"("Time / us"=w411) -> ("Time / s"=w410:dbl)  [unwired: 4 in]
        n145 = call "us_s_converter.vi"("Time / us"=10.0) -> ("Time / s"=w408:dbl)  [unwired: 4 in]
        n146 = call-poly "Configure Chan Mode.vi"("Width (10 msec)"=w408, "Delay (10 msec)"=w410, "Channel (1:Chan A)"=w412, "error in (no error)"=w415, "VISA resource name"=w416) -> ("error out"=w413:errorcluster, "VISA resource name out"=w414:refnum<visa-resource-name>)  [unwired: 5 in]
      }
      event "stop": Value Change {
        n147 = event-data() -> ()  [unwired: 1 in, 6 out]
      }
    }
  }
  n148 = Current VI's Path() -> (path=w20:path)
  n149 = Build Array("Target rotation / V", "Target translation / V", "Float / V", w52, w52, w52) -> (w23:dbl[])
  n150 = Current VI's Path() -> (path=w31:path)
  n151 = Build Array("Ref Repeller / V", "Ref Extractor / V", "Ref Gnd / V", "Einzel C 2 / V", "Deflection Plate  1 / V", "Deflection Plate  2 / V 2", "R1 / V 2", "R2 / V", "MCP") -> (w1:dbl[])
  n152 = Current VI's Path() -> (path=w9:path)
  n153 = call "DC_CNTRL_initialise_and_get_max_potentials.vi"("Device Index"=u32 0, "Box Number"=w13, "Input Potentials"=w12, "Current VI Path"=w20, "error in (no error)"=errorcluster {"status"=FALSE, "code"=0, "source"=""}) -> ("Handle out"=w19:u64, "Current Module"=w17:i32, "Max Range Array"=w18:dbl[], "error out"=w16:errorcluster)  [unwired: 7 in]
  n154 = call "DC_CNTRL_initialise_and_get_max_potentials.vi"("Device Index"=u32 2, "Box Number"=w24, "Input Potentials"=w23, "Current VI Path"=w31, "error in (no error)"=errorcluster {"status"=FALSE, "code"=0, "source"=""}) -> ("Handle out"=w30:u64, "Current Module"=w28:i32, "Max Range Array"=w29:dbl[], "error out"=w27:errorcluster)  [unwired: 7 in]
  n155 = call "DC_CNTRL_initialise_and_get_max_potentials.vi"("Device Index"=u32 4, "Box Number"=w2, "Input Potentials"=w1, "Current VI Path"=w9, "error in (no error)"=errorcluster {"status"=FALSE, "code"=0, "source"=""}) -> ("Handle out"=w8:u64, "Current Module"=w6:i32, "Max Range Array"=w7:dbl[], "error out"=w5:errorcluster)  [unwired: 7 in]
  n156 = while {
    tunnel: w19 -> [w428]
    tunnel: w18 -> [w427]
    tunnel: w16 -> [w425]
    shift-right: [w424] -> _
    shift-left: w17 -> [w426]
    tunnel: [w423] -> w15
    tunnel: [w422] -> w14
    tunnel: w13 -> [w420]
    stop <- w421 stop-if-true
    n157 = event shown="[0] \"Einzel A 1+3 / V\": Value Change" {
      selector: _ -> [_ _ _ _ _ _ _ _ _]
      dyn-events: _ -> [_ _ _ _ _ _ _ _ _]
      timeout: _ -> [_ _ _ _ _ _ _ _ _]
      tunnel: w428 -> [w440 w452 w464 w476 w488 w500 w512 w524 w527]
      tunnel: w427 -> [w437 w449 w461 w473 w485 w497 w509 w521 _]
      tunnel: w426 -> [w436 w448 w460 w472 w484 w496 w508 w520 w525]
      tunnel: w425 -> [w435 w447 w459 w471 w483 w495 w507 w519 w526]
      tunnel: [w434 w446 w458 w470 w482 w494 w506 w518 w525] -> w424
      tunnel: [w431 w443 w455 w467 w479 w491 w503 w515 w527] -> w423
      tunnel: [w430 w442 w454 w466 w478 w490 w502 w514 w526] -> w422
      tunnel: [_ _ _ _ _ _ _ _ TRUE] -> w421
      tunnel: w420 -> [w429 w441 w453 w465 w477 w489 w501 w513 _]
      event "Einzel A 1+3 / V": Value Change {
        w432 = u16 0 items=["0", "1", "2", "3", "4", "5", "6", "7"] ("Desired Module Number")
        n158 = event-data() -> ("OldVal"=w439:dbl, "NewVal"=w438:dbl)  [unwired: 1 in, 4 out]
        n159 = Index Array(array=w437, index=w432) -> (element=w433:dbl)
        n160 = call "DC_CNTRL_fast_select_module_and_change_potential.vi"("Handle in"=w440, "Current Potential (V)"=w439, "Target Potential (V)"=w438, "Max Potential (V)"=w433, "Box Number"=w429, "Current Module Number"=w436, "Desired Module Number"=w432, "error in (no error)"=w435) -> ("Handle out"=w431:u64, "Current Module Number Out"=w434:u16, "error out"=w430:errorcluster)  [unwired: 5 in]
      }
      event "Einzel A 2 / V": Value Change {
        w444 = u16 1 items=["0", "1", "2", "3", "4", "5", "6", "7"] ("Desired Module Number")
        n161 = event-data() -> ("OldVal"=w451:dbl, "NewVal"=w450:dbl)  [unwired: 1 in, 4 out]
        n162 = Index Array(array=w449, index=w444) -> (element=w445:dbl)
        n163 = call "DC_CNTRL_fast_select_module_and_change_potential.vi"("Handle in"=w452, "Current Potential (V)"=w451, "Target Potential (V)"=w450, "Max Potential (V)"=w445, "Box Number"=w441, "Current Module Number"=w448, "Desired Module Number"=w444, "error in (no error)"=w447) -> ("Handle out"=w443:u64, "Current Module Number Out"=w446:u16, "error out"=w442:errorcluster)  [unwired: 5 in]
      }
      event "Deceleration Float / V": Value Change {
        w456 = u16 2 items=["0", "1", "2", "3", "4", "5", "6", "7"] ("Desired Module Number")
        n164 = event-data() -> ("OldVal"=w463:dbl, "NewVal"=w462:dbl)  [unwired: 1 in, 4 out]
        n165 = Index Array(array=w461, index=w456) -> (element=w457:dbl)
        n166 = call "DC_CNTRL_fast_select_module_and_change_potential.vi"("Handle in"=w464, "Current Potential (V)"=w463, "Target Potential (V)"=w462, "Max Potential (V)"=w457, "Box Number"=w453, "Current Module Number"=w460, "Desired Module Number"=w456, "error in (no error)"=w459) -> ("Handle out"=w455:u64, "Current Module Number Out"=w458:u16, "error out"=w454:errorcluster)  [unwired: 5 in]
      }
      event "Einzel B 2 / V": Value Change {
        w468 = u16 3 items=["0", "1", "2", "3", "4", "5", "6", "7"] ("Desired Module Number")
        n167 = event-data() -> ("OldVal"=w475:dbl, "NewVal"=w474:dbl)  [unwired: 1 in, 4 out]
        n168 = Index Array(array=w473, index=w468) -> (element=w469:dbl)
        n169 = call "DC_CNTRL_fast_select_module_and_change_potential.vi"("Handle in"=w476, "Current Potential (V)"=w475, "Target Potential (V)"=w474, "Max Potential (V)"=w469, "Box Number"=w465, "Current Module Number"=w472, "Desired Module Number"=w468, "error in (no error)"=w471) -> ("Handle out"=w467:u64, "Current Module Number Out"=w470:u16, "error out"=w466:errorcluster)  [unwired: 5 in]
      }
      event "Def Top / V": Value Change {
        w480 = u16 4 items=["0", "1", "2", "3", "4", "5", "6", "7"] ("Desired Module Number")
        n170 = event-data() -> ("OldVal"=w487:dbl, "NewVal"=w486:dbl)  [unwired: 1 in, 4 out]
        n171 = Index Array(array=w485, index=w480) -> (element=w481:dbl)
        n172 = call "DC_CNTRL_fast_select_module_and_change_potential.vi"("Handle in"=w488, "Current Potential (V)"=w487, "Target Potential (V)"=w486, "Max Potential (V)"=w481, "Box Number"=w477, "Current Module Number"=w484, "Desired Module Number"=w480, "error in (no error)"=w483) -> ("Handle out"=w479:u64, "Current Module Number Out"=w482:u16, "error out"=w478:errorcluster)  [unwired: 5 in]
      }
      event "Def Bottom / V": Value Change {
        w492 = u16 5 items=["0", "1", "2", "3", "4", "5", "6", "7"] ("Desired Module Number")
        n173 = event-data() -> ("OldVal"=w499:dbl, "NewVal"=w498:dbl)  [unwired: 1 in, 4 out]
        n174 = Index Array(array=w497, index=w492) -> (element=w493:dbl)
        n175 = call "DC_CNTRL_fast_select_module_and_change_potential.vi"("Handle in"=w500, "Current Potential (V)"=w499, "Target Potential (V)"=w498, "Max Potential (V)"=w493, "Box Number"=w489, "Current Module Number"=w496, "Desired Module Number"=w492, "error in (no error)"=w495) -> ("Handle out"=w491:u64, "Current Module Number Out"=w494:u16, "error out"=w490:errorcluster)  [unwired: 5 in]
      }
      event "Def Left / V": Value Change {
        w504 = u16 6 items=["0", "1", "2", "3", "4", "5", "6", "7"] ("Desired Module Number")
        n176 = event-data() -> ("OldVal"=w511:dbl, "NewVal"=w510:dbl)  [unwired: 1 in, 4 out]
        n177 = Index Array(array=w509, index=w504) -> (element=w505:dbl)
        n178 = call "DC_CNTRL_fast_select_module_and_change_potential.vi"("Handle in"=w512, "Current Potential (V)"=w511, "Target Potential (V)"=w510, "Max Potential (V)"=w505, "Box Number"=w501, "Current Module Number"=w508, "Desired Module Number"=w504, "error in (no error)"=w507) -> ("Handle out"=w503:u64, "Current Module Number Out"=w506:u16, "error out"=w502:errorcluster)  [unwired: 5 in]
      }
      event "Def Right / V": Value Change {
        w516 = u16 7 items=["0", "1", "2", "3", "4", "5", "6", "7"] ("Desired Module Number")
        n179 = event-data() -> ("OldVal"=w523:dbl, "NewVal"=w522:dbl)  [unwired: 1 in, 4 out]
        n180 = Index Array(array=w521, index=w516) -> (element=w517:dbl)
        n181 = call "DC_CNTRL_fast_select_module_and_change_potential.vi"("Handle in"=w524, "Current Potential (V)"=w523, "Target Potential (V)"=w522, "Max Potential (V)"=w517, "Box Number"=w513, "Current Module Number"=w520, "Desired Module Number"=w516, "error in (no error)"=w519) -> ("Handle out"=w515:u64, "Current Module Number Out"=w518:u16, "error out"=w514:errorcluster)  [unwired: 5 in]
      }
      event "stop": Value Change {
        n182 = event-data() -> ()  [unwired: 1 in, 6 out]
      }
    }
  }
  n183 = while {
    tunnel: w30 -> [w537]
    tunnel: w29 -> [w536]
    tunnel: w27 -> [w534]
    shift-right: [w533] -> _
    shift-left: w28 -> [w535]
    tunnel: [w532] -> w26
    tunnel: [w531] -> w25
    tunnel: w24 -> [w529]
    stop <- w530 stop-if-true
    n184 = event shown="[0] \"Target rotation / V\": Value Change" {
      selector: _ -> [_ _ _ _]
      dyn-events: _ -> [_ _ _ _]
      timeout: _ -> [_ _ _ _]
      tunnel: w537 -> [w549 w561 w573 w577]
      tunnel: w536 -> [w546 w558 w570 _]
      tunnel: w535 -> [w545 w557 w569 w575]
      tunnel: w534 -> [w544 w556 w568 w576]
      tunnel: [w543 w555 w567 w575] -> w533
      tunnel: [w540 w552 w564 w577] -> w532
      tunnel: [w539 w551 w563 w576] -> w531
      tunnel: [_ _ _ "stop"] -> w530
      tunnel: w529 -> [w538 w550 w562 _]
      event "Target rotation / V": Value Change {
        w541 = u16 0 items=["0", "1", "2", "3", "4", "5", "6", "7"] ("Desired Module Number")
        n185 = event-data() -> ("OldVal"=w548:dbl, "NewVal"=w547:dbl)  [unwired: 1 in, 4 out]
        n186 = Index Array(array=w546, index=w541) -> (element=w542:dbl)
        n187 = call "DC_CNTRL_fast_select_module_and_change_potential.vi"("Handle in"=w549, "Current Potential (V)"=w548, "Target Potential (V)"=w547, "Max Potential (V)"=w542, "Box Number"=w538, "Current Module Number"=w545, "Desired Module Number"=w541, "error in (no error)"=w544) -> ("Handle out"=w540:u64, "Current Module Number Out"=w543:u16, "error out"=w539:errorcluster)  [unwired: 5 in]
      }
      event "Target translation / V": Value Change {
        w553 = u16 1 items=["0", "1", "2", "3", "4", "5", "6", "7"] ("Desired Module Number")
        n188 = event-data() -> ("OldVal"=w560:dbl, "NewVal"=w559:dbl)  [unwired: 1 in, 4 out]
        n189 = Index Array(array=w558, index=w553) -> (element=w554:dbl)
        n190 = call "DC_CNTRL_fast_select_module_and_change_potential.vi"("Handle in"=w561, "Current Potential (V)"=w560, "Target Potential (V)"=w559, "Max Potential (V)"=w554, "Box Number"=w550, "Current Module Number"=w557, "Desired Module Number"=w553, "error in (no error)"=w556) -> ("Handle out"=w552:u64, "Current Module Number Out"=w555:u16, "error out"=w551:errorcluster)  [unwired: 5 in]
      }
      event "Float / V": Value Change {
        w565 = u16 2 items=["0", "1", "2", "3", "4", "5", "6", "7"] ("Desired Module Number")
        n191 = event-data() -> ("OldVal"=w572:dbl, "NewVal"=w571:dbl)  [unwired: 1 in, 4 out]
        n192 = Index Array(array=w570, index=w565) -> (element=w566:dbl)
        n193 = call "DC_CNTRL_fast_select_module_and_change_potential.vi"("Handle in"=w573, "Current Potential (V)"=w572, "Target Potential (V)"=w571, "Max Potential (V)"=w566, "Box Number"=w562, "Current Module Number"=w569, "Desired Module Number"=w565, "error in (no error)"=w568) -> ("Handle out"=w564:u64, "Current Module Number Out"=w567:u16, "error out"=w563:errorcluster)  [unwired: 5 in]
      }
      event "stop": Value Change {
        (unwired) TRUE ("last element? (F)")
        n194 = event-data() -> ()  [unwired: 1 in, 6 out]
      }
    }
  }
  n195 = while {
    tunnel: w8 -> [w586]
    tunnel: w7 -> [w585]
    tunnel: w5 -> [w583]
    shift-right: [w582] -> _
    shift-left: w6 -> [w584]
    tunnel: [w581] -> w4
    tunnel: [w580] -> w3
    tunnel: w2 -> [w578]
    stop <- w579 stop-if-true
    n196 = event shown="[0] \"Ref Repeller / V\": Value Change" {
      selector: _ -> [_ _ _ _ _ _ _ _ _ _]
      dyn-events: _ -> [_ _ _ _ _ _ _ _ _ _]
      timeout: _ -> [_ _ _ _ _ _ _ _ _ _]
      tunnel: w586 -> [w598 w610 w622 w634 w646 w658 w670 w682 w694 w697]
      tunnel: w585 -> [w595 w607 w619 w631 w643 w655 w667 w679 w691 _]
      tunnel: w584 -> [w594 w606 w618 w630 w642 w654 w666 w678 w690 w695]
      tunnel: w583 -> [w593 w605 w617 w629 w641 w653 w665 w677 w689 w696]
      tunnel: [w592 w604 w616 w628 w640 w652 w664 w676 w688 w695] -> w582
      tunnel: [w589 w601 w613 w625 w637 w649 w661 w673 w685 w697] -> w581
      tunnel: [w588 w600 w612 w624 w636 w648 w660 w672 w684 w696] -> w580
      tunnel: [_ _ _ _ _ _ _ _ _ TRUE] -> w579
      tunnel: w578 -> [w587 w599 w611 w623 w635 w647 w659 w671 w683 _]
      event "Ref Repeller / V": Value Change {
        w590 = u16 0 items=["0", "1", "2", "3", "4", "5", "6", "7"] ("Desired Module Number")
        n197 = event-data() -> ("OldVal"=w597:dbl, "NewVal"=w596:dbl)  [unwired: 1 in, 4 out]
        n198 = Index Array(array=w595, index=w590) -> (element=w591:dbl)
        n199 = call "DC_CNTRL_fast_select_module_and_change_potential.vi"("Handle in"=w598, "Current Potential (V)"=w597, "Target Potential (V)"=w596, "Max Potential (V)"=w591, "Box Number"=w587, "Current Module Number"=w594, "Desired Module Number"=w590, "error in (no error)"=w593) -> ("Handle out"=w589:u64, "Current Module Number Out"=w592:u16, "error out"=w588:errorcluster)  [unwired: 5 in]
      }
      event "Ref Extractor / V": Value Change {
        w602 = u16 1 items=["0", "1", "2", "3", "4", "5", "6", "7"] ("Desired Module Number")
        n200 = event-data() -> ("OldVal"=w609:dbl, "NewVal"=w608:dbl)  [unwired: 1 in, 4 out]
        n201 = Index Array(array=w607, index=w602) -> (element=w603:dbl)
        n202 = call "DC_CNTRL_fast_select_module_and_change_potential.vi"("Handle in"=w610, "Current Potential (V)"=w609, "Target Potential (V)"=w608, "Max Potential (V)"=w603, "Box Number"=w599, "Current Module Number"=w606, "Desired Module Number"=w602, "error in (no error)"=w605) -> ("Handle out"=w601:u64, "Current Module Number Out"=w604:u16, "error out"=w600:errorcluster)  [unwired: 5 in]
      }
      event "Ref Gnd / V": Value Change {
        w614 = u16 2 items=["0", "1", "2", "3", "4", "5", "6", "7"] ("Desired Module Number")
        n203 = event-data() -> ("OldVal"=w621:dbl, "NewVal"=w620:dbl)  [unwired: 1 in, 4 out]
        n204 = Index Array(array=w619, index=w614) -> (element=w615:dbl)
        n205 = call "DC_CNTRL_fast_select_module_and_change_potential.vi"("Handle in"=w622, "Current Potential (V)"=w621, "Target Potential (V)"=w620, "Max Potential (V)"=w615, "Box Number"=w611, "Current Module Number"=w618, "Desired Module Number"=w614, "error in (no error)"=w617) -> ("Handle out"=w613:u64, "Current Module Number Out"=w616:u16, "error out"=w612:errorcluster)  [unwired: 5 in]
      }
      event "Einzel C 2 / V": Value Change {
        w626 = u16 3 items=["0", "1", "2", "3", "4", "5", "6", "7"] ("Desired Module Number")
        n206 = event-data() -> ("OldVal"=w633:dbl, "NewVal"=w632:dbl)  [unwired: 1 in, 4 out]
        n207 = Index Array(array=w631, index=w626) -> (element=w627:dbl)
        n208 = call "DC_CNTRL_fast_select_module_and_change_potential.vi"("Handle in"=w634, "Current Potential (V)"=w633, "Target Potential (V)"=w632, "Max Potential (V)"=w627, "Box Number"=w623, "Current Module Number"=w630, "Desired Module Number"=w626, "error in (no error)"=w629) -> ("Handle out"=w625:u64, "Current Module Number Out"=w628:u16, "error out"=w624:errorcluster)  [unwired: 5 in]
      }
      event "Deflection Plate  1 / V": Value Change {
        w638 = u16 4 items=["0", "1", "2", "3", "4", "5", "6", "7"] ("Desired Module Number")
        n209 = event-data() -> ("OldVal"=w645:dbl, "NewVal"=w644:dbl)  [unwired: 1 in, 4 out]
        n210 = Index Array(array=w643, index=w638) -> (element=w639:dbl)
        n211 = call "DC_CNTRL_fast_select_module_and_change_potential.vi"("Handle in"=w646, "Current Potential (V)"=w645, "Target Potential (V)"=w644, "Max Potential (V)"=w639, "Box Number"=w635, "Current Module Number"=w642, "Desired Module Number"=w638, "error in (no error)"=w641) -> ("Handle out"=w637:u64, "Current Module Number Out"=w640:u16, "error out"=w636:errorcluster)  [unwired: 5 in]
      }
      event "Deflection Plate  2 / V 2": Value Change {
        w650 = u16 5 items=["0", "1", "2", "3", "4", "5", "6", "7"] ("Desired Module Number")
        n212 = event-data() -> ("OldVal"=w657:dbl, "NewVal"=w656:dbl)  [unwired: 1 in, 4 out]
        n213 = Index Array(array=w655, index=w650) -> (element=w651:dbl)
        n214 = call "DC_CNTRL_fast_select_module_and_change_potential.vi"("Handle in"=w658, "Current Potential (V)"=w657, "Target Potential (V)"=w656, "Max Potential (V)"=w651, "Box Number"=w647, "Current Module Number"=w654, "Desired Module Number"=w650, "error in (no error)"=w653) -> ("Handle out"=w649:u64, "Current Module Number Out"=w652:u16, "error out"=w648:errorcluster)  [unwired: 5 in]
      }
      event "R1 / V 2": Value Change {
        w662 = u16 6 items=["0", "1", "2", "3", "4", "5", "6", "7"] ("Desired Module Number")
        n215 = event-data() -> ("OldVal"=w669:dbl, "NewVal"=w668:dbl)  [unwired: 1 in, 4 out]
        n216 = Index Array(array=w667, index=w662) -> (element=w663:dbl)
        n217 = call "DC_CNTRL_fast_select_module_and_change_potential.vi"("Handle in"=w670, "Current Potential (V)"=w669, "Target Potential (V)"=w668, "Max Potential (V)"=w663, "Box Number"=w659, "Current Module Number"=w666, "Desired Module Number"=w662, "error in (no error)"=w665) -> ("Handle out"=w661:u64, "Current Module Number Out"=w664:u16, "error out"=w660:errorcluster)  [unwired: 5 in]
      }
      event "R2 / V": Value Change {
        w674 = u16 7 items=["0", "1", "2", "3", "4", "5", "6", "7"] ("Desired Module Number")
        n218 = event-data() -> ("OldVal"=w681:dbl, "NewVal"=w680:dbl)  [unwired: 1 in, 4 out]
        n219 = Index Array(array=w679, index=w674) -> (element=w675:dbl)
        n220 = call "DC_CNTRL_fast_select_module_and_change_potential.vi"("Handle in"=w682, "Current Potential (V)"=w681, "Target Potential (V)"=w680, "Max Potential (V)"=w675, "Box Number"=w671, "Current Module Number"=w678, "Desired Module Number"=w674, "error in (no error)"=w677) -> ("Handle out"=w673:u64, "Current Module Number Out"=w676:u16, "error out"=w672:errorcluster)  [unwired: 5 in]
      }
      event "MCP": Value Change {
        w686 = u16 8 items=["0", "1", "2", "3", "4", "5", "6", "7", "8"] ("Desired Module Number")
        n221 = event-data() -> ("OldVal"=w693:dbl, "NewVal"=w692:dbl)  [unwired: 1 in, 4 out]
        n222 = Index Array(array=w691, index=w686) -> (element=w687:dbl)
        n223 = call "DC_CNTRL_fast_select_module_and_change_potential.vi"("Handle in"=w694, "Current Potential (V)"=w693, "Target Potential (V)"=w692, "Max Potential (V)"=w687, "Box Number"=w683, "Current Module Number"=w690, "Desired Module Number"=w686, "error in (no error)"=w689) -> ("Handle out"=w685:u64, "Current Module Number Out"=w688:u16, "error out"=w684:errorcluster)  [unwired: 5 in]
      }
      event "stop": Value Change {
        n224 = event-data() -> ()  [unwired: 1 in, 6 out]
      }
    }
  }
  n225 = call "FT_Close_Device_64bit.vi"("Handle"=w4, "error in (no error)"=w3) -> ()  [unwired: 12 in, 2 out]
  n226 = call "FT_Close_Device_64bit.vi"("Handle"=w15, "error in (no error)"=w14) -> ()  [unwired: 12 in, 2 out]
  n227 = call "Close.vi"("error in (no error)"=w56, "VISA resource name"=w57) -> ()  [unwired: 9 in, 1 out]
  n228 = call "FT_Close_Device_64bit.vi"("Handle"=w26, "error in (no error)"=w25) -> ()  [unwired: 12 in, 2 out]
